vi "UTILITY Local.vi"() -> (2 "Local?":bool)   [LabVIEW 2019]
panel:
  out "call chain":string[](array[string])
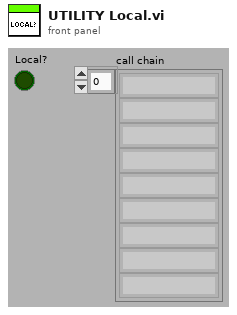
[diagram p1: front panel]
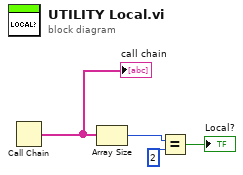
[diagram p0: block diagram]
diagram:
  n1 = Call Chain() -> (call chain=w2:string[])
  "call chain" <- w2
  n2 = Array Size(array=w2) -> (size(s)=w3:i32)
  n3 = Equal?(x=w3, y=2) -> (x = y?=→"Local?":bool)
